vi "ief_put_single_output.vi"(3 "error in (no error)":errorcluster, 4 "Single Output State":bool, 5 "Single Output Number":u16=1 min=1 max=1024, 6 "Tagprefix in":refnum<k21>) -> (0 "error out (no error)":errorcluster, 1 "Single Output State Out":bool, 2 "Tagprefix out":refnum<k21>)   [LabVIEW 2015, in "IEF Werner.lvlib"]
doc: "The VI sets the single output state of the chosen single output to the specified state. Furthermore It returns the present state of the chosen single output. If the command was executed correctly the single output state is equal to the single input state.\n\nSingle Output Number Range:\n0001 - 0400, hex\n1 - 1024, dec\n\nSingle Output State Range: Boolean"
uses:
  IEF Werner.lvlib
panel:
  # "IEF Put Single Output"
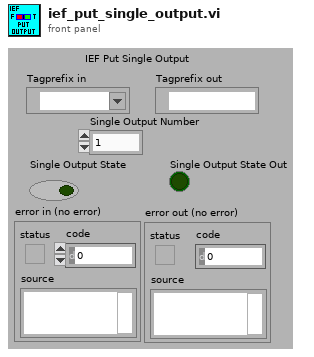
[diagram p1: front panel]
types:
  T1 = typedef "Semaphore RefNum" = refnum<k1>
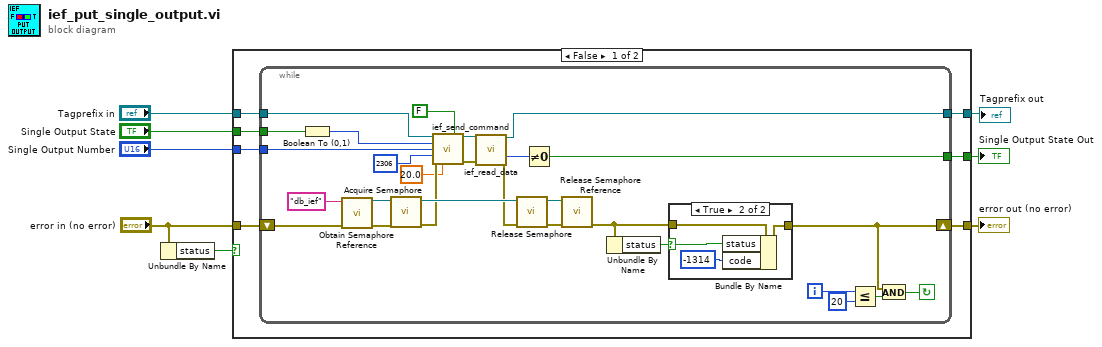
[diagram p0: block diagram]
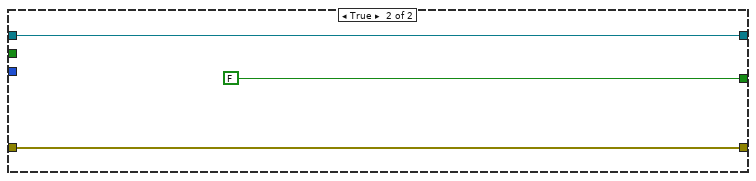
[diagram p3: hidden frame]
diagram:
  n1 = Unbundle By Name("error in (no error)") -> ("status"=w4:bool)
  n2 = case shown="False" w4 {
    tunnel: "Single Output State" -> [w15 _]
    tunnel: "Single Output Number" -> [w14 _]
    tunnel: "error in (no error)" -> [w11 w51]
    tunnel: [w13 w51] -> w6
    tunnel: [w12 FALSE] -> w3
    tunnel: "Tagprefix in" -> [w10 w50]
    tunnel: [w9 w50] -> w1
    frame False {
      n3 = while {
        tunnel: w15 -> [w41]
        tunnel: w14 -> [w40]
        tunnel: [w36] -> w12
        shift-right: [w16] -> w13
        shift-left: w11 -> [w28]
        tunnel: w10 -> [w24]
        tunnel: [w22] -> w9
        i -> [w18]
        stop <- w17 continue-if-true
        n4 = Boolean To (0,1)(Boolean=w41) -> (0, 1=w35:i16)
        n5 = call <vilib>:"Obtain Semaphore Reference.vi"("error in (no error)"=w28, "name (unnamed)"="db_ief") -> ("error out"=w32:errorcluster, "semaphore"=w33:T1)  [unwired: 3 in, 1 out]
        n6 = call <vilib>:"Acquire Semaphore.vi"("error in (no error)"=w32, "semaphore"=w33) -> ("error out"=w27:errorcluster, "semaphore out"=w31:T1)  [unwired: 3 in, 1 out]
        n7 = call "ief_send_command.vi"("Tagprefix in"=w24, "Command datum of type real"=FALSE, "Command datum"=w35, "Command parameter"=w40, "Command code"=u16 2306, "error in (no error)"=w27, "time out [s]"=20.0) -> ("Tagprefix out"=w23:refnum<k21>, "error out (no error)"=w39:errorcluster)  [unwired: 3 in, 4 out]
        n8 = call "ief_read_data.vi"("Tagprefix in"=w23, "error in (no error)"=w39) -> ("Tagprefix out"=w22:refnum<k21>, "value uint 16"=w37:u16, "error out (no error)"=w26:errorcluster)  [unwired: 7 in, 4 out]
        n9 = call <vilib>:"Release Semaphore.vi"("error in (no error)"=w26, "semaphore"=w31) -> ("error out"=w30:errorcluster, "semaphore out"=w29:T1)  [unwired: 4 in]
        n10 = Not Equal To 0?(x=w37) -> (x != 0?=w36:bool)
        n11 = call <vilib>:"Release Semaphore Reference.vi"("error in (no error)"=w30, "semaphore"=w29) -> ("error out"=w25:errorcluster)  [unwired: 8 in, 1 out]
        n12 = Unbundle By Name(w25) -> ("status"=w38:bool)
        n13 = case shown="True" w38 {
          selector: w38 -> [_ w45]
          tunnel: [w44 w47] -> w16
          tunnel: w25 -> [w44 w48]
          frame False {
          }
          frame True {
            n14 = Bundle By Name(cluster=w48, "status"=w45, "code"=-1314) -> (w47:errorcluster)
          }
        }
        n15 = Less Or Equal?(x=w18, y=20) -> (x <= y?=w19:bool)
        n16 = And(x=w16, y=w19) -> (x .and. y?=w17:bool)
      }
    }
    frame True {
    }
  }
  "error out (no error)" <- w6
  "Single Output State Out" <- w3
  "Tagprefix out" <- w1
